vi "Class Name.vi"() -> (3 "class name":string)   [LabVIEW 2017, in "DSF Core.lvlib" / "Dispatcher Interface.lvclass"]
uses:
  Dispatcher Interface.lvclass
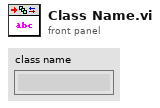
[diagram p1: front panel]
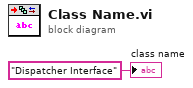
[diagram p0: block diagram]
diagram:
  "class name" <- "Dispatcher Interface" ("class name")
